vi "Flush_Ga_00.vi"() -> ()   [LabVIEW 2011]
panel:
  in  "stop":bool
  out "Numeric":i32 caption="iteration"
  in  "Iterations":i32=20
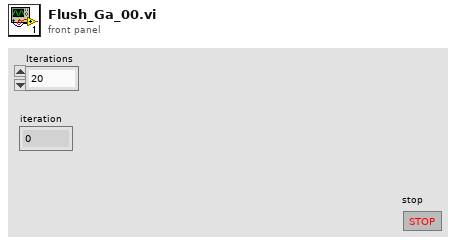
[diagram p1: front panel]
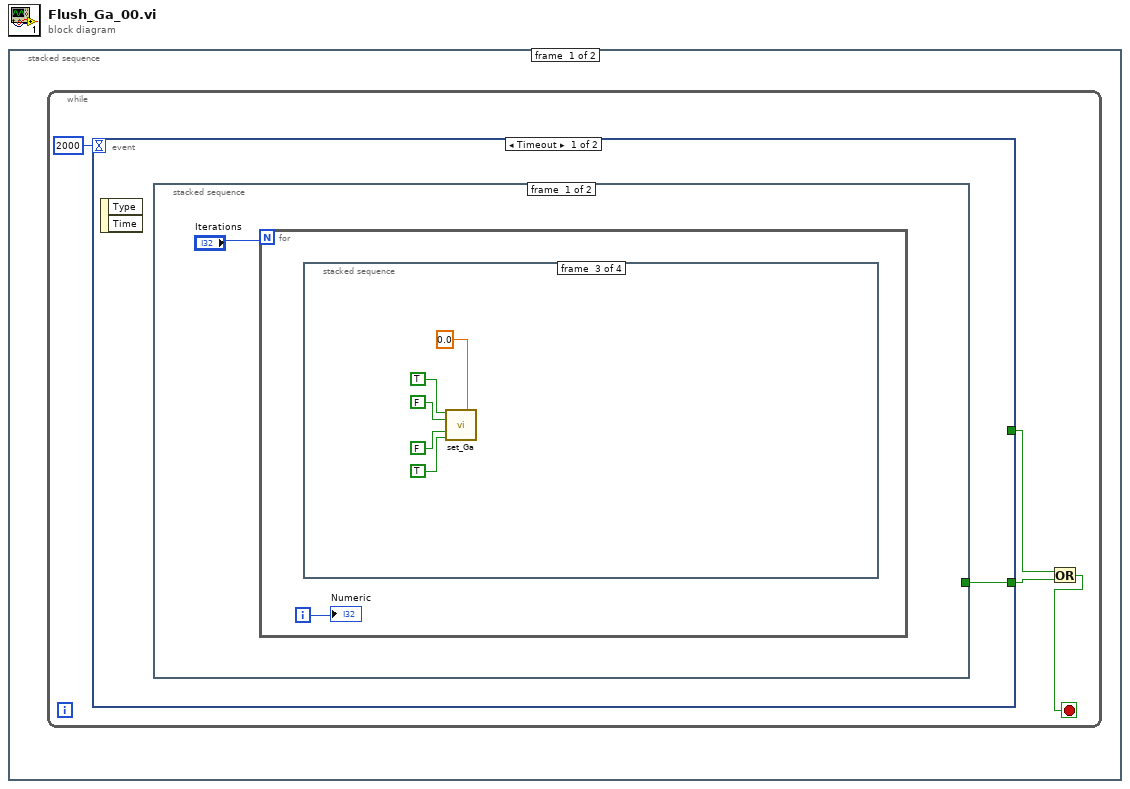
[diagram p0: block diagram]
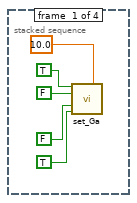
[diagram p2: hidden frame]
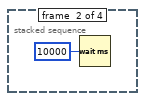
[diagram p3: hidden frame]
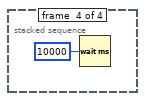
[diagram p4: hidden frame]
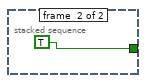
[diagram p5: hidden frame]
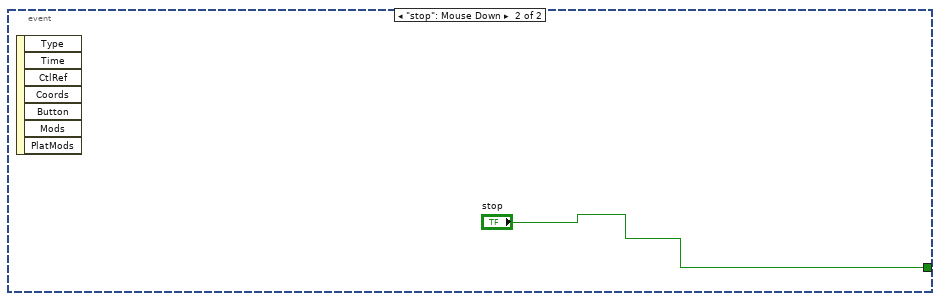
[diagram p6: hidden frame]
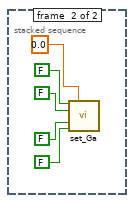
[diagram p7: hidden frame]
diagram:
  n1 = stacked-sequence {
    frame #0 {
      n2 = while {
        stop <- w2 stop-if-true
        n3 = event shown="[0] Timeout" {
          selector: _ -> [_ _]
          dyn-events: _ -> [_ _]
          timeout: 2000 -> [_ _]
          tunnel: [_ "stop"] -> w3
          tunnel: [w5 _] -> w4
          event Timeout {
            n4 = event-data() -> ()  [unwired: 1 in, 2 out]
            n5 = stacked-sequence {
              tunnel: [_ TRUE] -> w5
              frame #0 {
                n6 = for {
                  N: "Iterations" -> [_]
                  i -> [w7]
                  n7 = stacked-sequence {
                    frame #0 {
                      n8 = call "set_Ga.vi"("Ga Active"=TRUE ("As_Gas Active"), "Ga Flow 1"=10.0 ("As_Gas Flow"), "Ga Bubbler"=FALSE ("As_Gas In"), "Ga Run"=FALSE ("As_Gas Run"), "Ga Remote"=TRUE ("As_Gas Remote")) -> ()  [unwired: 11 in]
                    }
                    frame #1 {
                      n9 = Wait (ms)(milliseconds to wait=u32 10000) -> ()  [unwired: 1 out]
                    }
                    frame #2 {
                      n10 = call "set_Ga.vi"("Ga Active"=TRUE ("As_Gas Active"), "Ga Flow 1"=0.0 ("Ga Flow 3"), "Ga Bubbler"=FALSE ("As_Gas In"), "Ga Run"=FALSE ("As_Gas Run"), "Ga Remote"=TRUE ("As_Gas Remote")) -> ()  [unwired: 11 in]
                    }
                    frame #3 {
                      n11 = Wait (ms)(milliseconds to wait=u32 10000) -> ()  [unwired: 1 out]
                    }
                  }
                  "Numeric" <- w7
                }
              }
              frame #1 {
              }
            }
          }
          event "stop": Mouse Down {
            n12 = event-data() -> ()  [unwired: 1 in, 7 out]
          }
        }
        n13 = Or(x=w3, y=w4) -> (x .or. y?=w2:bool)
      }
    }
    frame #1 {
      n14 = call "set_Ga.vi"("Ga Active"=FALSE ("As_Gas Active"), "Ga Flow 3"=0.0 ("As_Gas Flow"), "Ga Bubbler"=FALSE ("As_Gas In"), "Ga Run"=FALSE ("As_Gas Run"), "Ga Remote"=FALSE ("As_Gas Remote")) -> ()  [unwired: 11 in]
    }
  }
